vi "MasterRobotModeController.vi"() -> (1 "FMS Robot Mode":T1, 2 "Auto Reset":bool, 3 "Robot is Autonomous":bool)   [LabVIEW 2020]
doc: "This state controller manages the Robot Mode and whether or not the robot is running autonomously. The robot will continue running autonomously after Autonomous Mode ends, until the driver touches the joystick during TeleOperated Mode or until/unless the FORCE HUMAN CONTROL override is flipped on the FRC 4265 Dashboard."
uses:
  <vilib>/Rock Robotics/WPI/DriverStation/WPI_DriverStationRobotMode2.ctl
  refnums.vi
  GRNF_Joystick.vi
  dsdata.vi
  constants3.vi
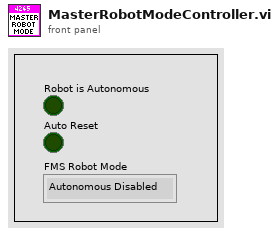
[diagram p1: front panel]
types:
  T1 = typedef "WPI_DriverStationRobotMode2.ctl" = enum16{"Autonomous Disabled", "Autonomous Enabled", "Teleop Disabled", "Teleop Enabled", "Disconnected", "Finish", "Test Disabled", "Test Enabled", "Emergency Stopped"}
  T2 = typedef "WPI_JoystickDevRef.ctl" = cluster{"Device":T3}
  T3 = typedef "WPI_JoystickDeviceEnum.ctl" = enum16{"USB 0", "USB 1", "USB 2", "USB 3", "USB 4", "USB 5"}
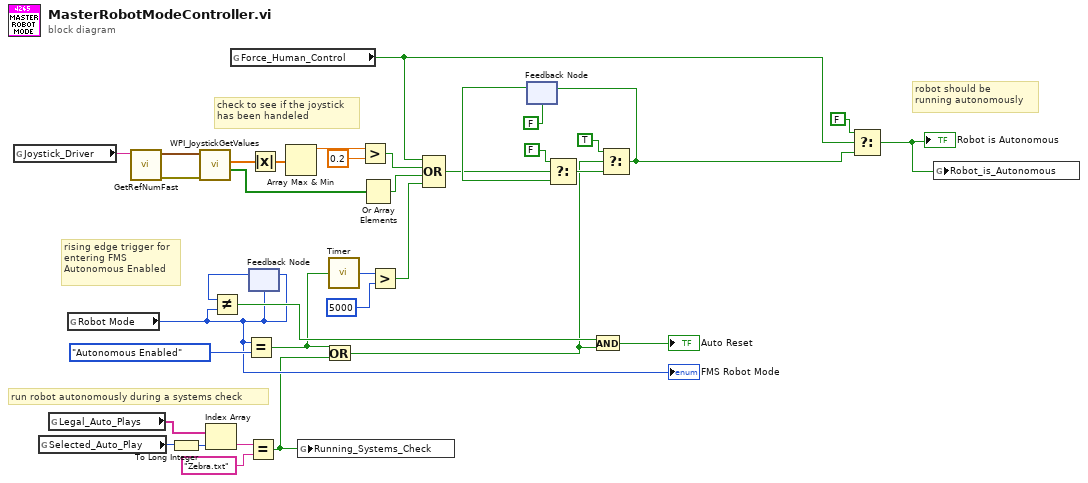
[diagram p0: block diagram]
diagram:
  # "run robot autonomously during a systems check"
  # "rising edge trigger for\nentering FMS\nAutonomous Enabled"
  # "robot should be\nrunning autonomously"
  # "check to see if the joystick \nhas been handeled"
  n1 = global read "refnums.vi" "Joystick_Driver"() -> (w34:string)
  n2 = global read "dsdata.vi" "Selected_Auto_Play"() -> (w7:u16)
  n3 = global read "constants3.vi" "Legal_Auto_Plays"() -> (w1:string[])
  n4 = global read "dsdata.vi" "Robot Mode"() -> (w16:T1)
  "FMS Robot Mode" <- w16
  n5 = call-poly "GetRefNumFast.vi"("RefNum Name"=w34) -> ("Error"=w35:errorcluster, "Device Reference"=w36:T2)  [unwired: 5 in]
  n6 = To Long Integer(number=w7) -> (32bit integer=w8:i32)
  n7 = call <vilib>:"WPI_JoystickGetValues.vi"("error in (no error)"=w35, "JoystickDevRef"=w36) -> ("Buttons"=w33:bool[], "Axes"=w32:dbl[])  [unwired: 5 in, 3 out]
  n8 = Index Array(array=w1, index=w8) -> (element=w6:string)
  n9 = global read "dsdata.vi" "Force_Human_Control"() -> (w12:bool)
  n10 = Equal?(x=w16, y=WPI_DriverStationRobotMode2."Autonomous Enabled" ("Robot Mode")) -> (x = y?=w3:bool)
  n11 = Equal?(x=w6, y="Zebra.txt") -> (x = y?=w2:bool)
  n12 = feedback #1(w16) -> (w23:T1)
  n13 = Not Equal?(x=w23, y=w16) -> (x != y?=w22:bool)
  n14 = feedback-in #1(w16) -> ()
  n15 = Absolute Value(x=w32) -> (abs(x)=w31:dbl[])
  n16 = Array Max & Min(array=w31) -> (max value=w30:dbl)  [unwired: 3 out]
  n17 = global write "dsdata.vi" "Running_Systems_Check"(w2) -> ()
  n18 = Or(x=w3, y=w2) -> (x .or. y?=w4:bool)
  n19 = call "Timer.vi"("Reset Timer"=w3) -> ("Time (ms)"=w11:u32)
  n20 = Greater?(x=w30, y=0.2) -> (0:w28:bool)
  n21 = Or Array Elements(Boolean array=w33) -> (logical OR=w27:bool)
  n22 = Greater?(x=w11, y=u32 5000) -> (0:w9:bool)
  n23 = Compound Arithmetic op=OR(w12, w28, w27, w9) -> (w17:bool)
  n24 = feedback #2(FALSE) -> (w18:bool)
  n25 = Select(t=FALSE, s=w17, f=w18) -> (s? t:f=w19:bool)
  n26 = And(x=w22, y=w4) -> (x .and. y?=→"Auto Reset":bool)
  n27 = Select(t=TRUE, s=w4, f=w19) -> (s? t:f=w14:bool)
  n28 = feedback-in #2(w14) -> ()
  n29 = Select(t=FALSE, s=w12, f=w14) -> (s? t:f=w13:bool)
  "Robot is Autonomous" <- w13
  n30 = global write "dsdata.vi" "Robot_is_Autonomous"(w13) -> ()
